vi "Power Train Test.vi"(4 "Sequence Context":T1) -> (0 "error out":errorcluster, 1 "Test Data":T2 {"Numeric Measurement" format="%.2f"})   [LabVIEW 2012]
uses:
  <vilib>/addons/TestStand/_TSLegacy.llb/LabVIEW Test - Test Data.ctl
  <vilib>/addons/TestStand/_TSLegacy.llb/LabVIEW Test - Sequence Context.ctl
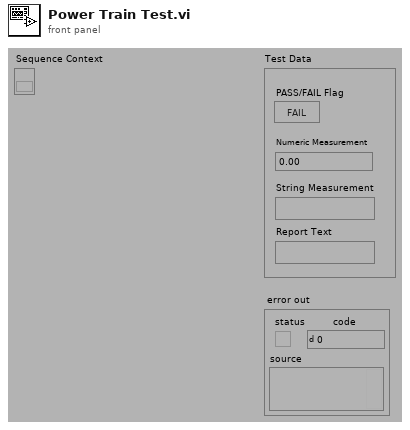
[diagram p1: front panel]
types:
  T1 = typedef "LabVIEW Test - Sequence Context.ctl" = refnum<k7>
  T2 = typedef "LabVIEW Test - Test Data.ctl" = cluster{"PASS/FAIL Flag":bool, "Numeric Measurement":dbl, "String Measurement":string, "Report Text":string}
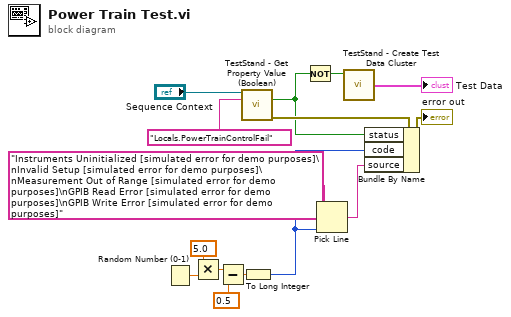
[diagram p0: block diagram]
diagram:
  n1 = Random Number (0-1)() -> (number: 0 to 1=w10:dbl)
  n2 = Multiply(x=5.0, y=w10) -> (x*y=w9:dbl)
  n3 = Subtract(x=w9, y=0.5 ("x")) -> (x-y=w8:dbl)
  n4 = call "TestStand - Get Property Value (Boolean).vi"("Sequence Context In"="Sequence Context", "Lookup String"="Locals.PowerTrainControlFail") -> ("Value"=w4:bool, "error out"=w6:errorcluster)  [unwired: 1 in, 11 out]
  n5 = To Long Integer(number=w8) -> (32bit integer=w2:i32)
  n6 = Not(x=w4) -> (.not. x?=w12:bool)
  n7 = Pick Line(multi-line string="Instruments Uninitialized [simulated error for demo purposes]\nInvalid Setup [simulated error for demo purposes]\nMeasurement Out of Range [simulated error for demo purposes]\nGPIB Read Error [simulated error for demo purposes]\nGPIB Write Error [simulated error for demo purposes]" ("Lookup String"), line index=w2) -> (output string=w1:string)  [unwired: 1 out]
  n8 = call "TestStand - Create Test Data Cluster.vi"("PASS/FAIL Flag"=w12) -> ("Test Data"=→"Test Data":T2)  [unwired: 3 in]
  n9 = Bundle By Name(cluster=w6, "status"=w4, "code"=w2, "source"=w1) -> (→"error out":errorcluster)
